vi "oa_Draw Grids and Plot for SCL Plot.vi"(5 "shaft center line settings":T3={"cartesian grid cosmetics"={"line color"=39168, "text color"=65280, "tick length(3)"=3, "crossing axes"=FALSE, "visible grid?"=TRUE}, "XY plot cosmetics"={"plot color"=16776960, "XY plot type"=enum."connected points", "baseline"=0.0}, "desired font(Application)"=enum."Application Font", "[user-specified font]"={"Font Name:"="", "Size"=0, "Strikeout?"=FALSE, "Italic?"=FALSE, "Underline?"=FALSE, "Outline?"=FALSE, "Shadow?"=FALSE, "Bold?"=FALSE}} {"XY plot cosmetics"."baseline" format="%0.2f"}, 6 "shaft rotating direction":u16(ring) items=["CCW", "CW"], 7 "picture \ndimensions (w,h)":cluster{"width":u32, "height":u32}, 8 "error in (no error)":errorcluster, 9 "scale":T1, 10 "DC Gap":cluster{"X":dbl[], "Y":dbl[]}[](array[cluster]) {"Y" format="%.2f"; "X" format="%.2f"}, 11 "picture":picture) -> (0 "error out":errorcluster, 1 "y scale factors":cluster{"a":dbl, "b":dbl, "log?":bool} {"b" format="%0.2f"; "a" format="%0.2f"}, 2 "x scale factors":cluster{"a":dbl, "b":dbl, "log?":bool} {"b" format="%0.2f"; "a" format="%0.2f"}, 3 "new picture":picture)   [LabVIEW 2017]
uses:
  <vilib>/picture/cartesn2.llb/XY Plot Type.ctl
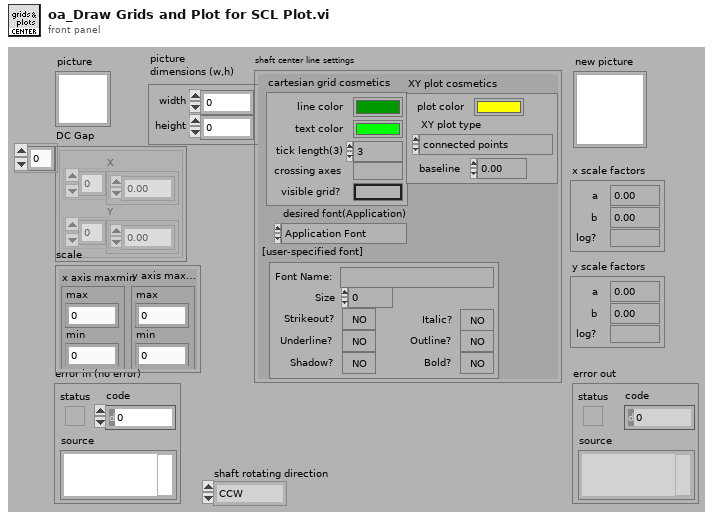
[diagram p1: front panel]
types:
  T1 = cluster{"x axis maxmin":cluster{"max":dbl, "min":dbl}, "y axis maxmin":cluster{"max":dbl, "min":dbl}}
  T2 = typedef "XY Plot Type.ctl" = enum16{"points", "squares", "circles", "connected points", "connected squares", "connected circles", "comb plot", "sized scatter plot", "sized-colored scatter plot", "min-max lines"}
  T3 = cluster{"cartesian grid cosmetics":cluster{"line color":u32, "text color":u32, "tick length(3)":i16, "crossing axes":bool, "visible grid?":bool}, "XY plot cosmetics":cluster{"plot color":u32, "XY plot type":T2, "baseline":dbl}, "desired font(Application)":enum16{"User-specified Font", "Application Font", "System Font", "Dialog Font"}, "[user-specified font]":cluster{"Font Name:":string, "Size":i16, "Strikeout?":bool, "Italic?":bool, "Underline?":bool, "Outline?":bool, "Shadow?":bool, "Bold?":bool}}
  T4 = cluster{"x minimum":dbl, "x maximum":dbl, "x log?":bool, "x precision":u8, "x format":enum8{"Decimal", "Scientific", "Engineering", "Binary", "Octal", "Hex"}, "y minimum":dbl, "y maximum":dbl, "y log?":bool, "y precision":u8, "y format":enum8{"Decimal", "Scientific", "Engineering", "Binary", "Octal", "Hex"}}
  T5 = enum8{"Decimal", "Scientific", "Engineering", "Binary", "Octal", "Hex"}
  T6 = cluster{"line color":u32, "text color":u32, "tick length(3)":i16, "crossing axes":bool, "visible grid?":bool}
  T7 = cluster{"plot color":u32, "XY plot type":T2, "baseline":dbl}
  T8 = enum16{"User-specified Font", "Application Font", "System Font", "Dialog Font"}
  T9 = cluster{"Font Name:":string, "Size":i16, "Strikeout?":bool, "Italic?":bool, "Underline?":bool, "Outline?":bool, "Shadow?":bool, "Bold?":bool}
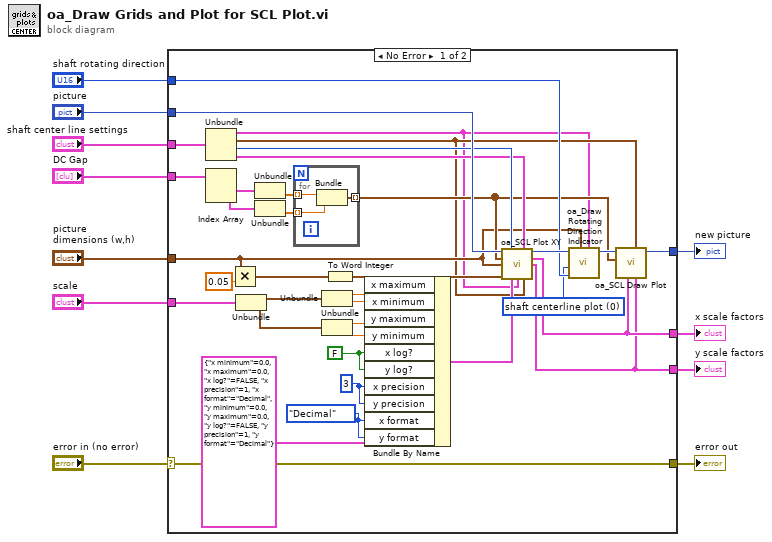
[diagram p0: block diagram]
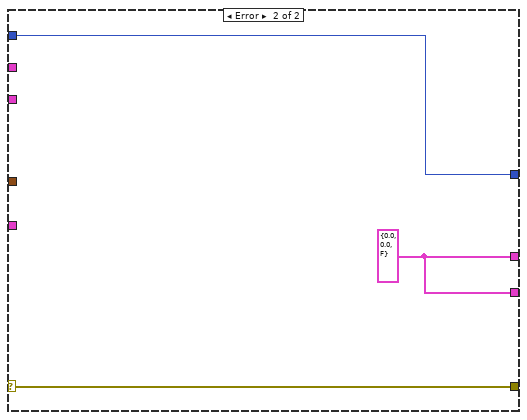
[diagram p2: hidden frame]
diagram:
  n1 = case shown="No Error" "error in (no error)" {
    selector: "error in (no error)" -> [w45 w53]
    tunnel: [w45 w53] -> w10
    tunnel: "picture" -> [w47 w52]
    tunnel: "shaft center line settings" -> [w46 _]
    tunnel: "picture \ndimensions (w,h)" -> [w17 _]
    tunnel: [w19 w52] -> w6
    tunnel: "DC Gap" -> [w44 _]
    tunnel: "scale" -> [w36 _]
    tunnel: "shaft rotating direction" -> [w21 _]
    tunnel: [w15 w51] -> w2
    tunnel: [w14 w51] -> w1
    frame No Error {
      w27 = T5."Decimal" ("x format")
      w28 = u8 3 ("x precision")
      w12 = u16 0 items=["shaft centerline plot", "polar plot"] ("plot type")
      w29 = FALSE ("x log?")
      n2 = Unbundle(w46) -> ("cartesian grid cosmetics"=w13:T6, "XY plot cosmetics"=w16:T7, "desired font(Application)"=w39:T8, "[user-specified font]"=w38:T9)
      n3 = Index Array(array=w44) -> (element #1=w43:cluster{"X":dbl[], "Y":dbl[]}, element #2=w42:cluster{"X":dbl[], "Y":dbl[]})  [unwired: 2 in]
      n4 = Multiply(x=w17, y=0.05) -> (x*y=w24:cluster{"width":dbl, "height":dbl})
      n5 = Unbundle(w36) -> ("x axis maxmin"=w35:cluster{"max":dbl, "min":dbl}, "y axis maxmin"=w33:cluster{"max":dbl, "min":dbl})
      n6 = Unbundle(w43) -> ("Y"=w41:dbl[])  [unwired: 1 out]
      n7 = Unbundle(w42) -> ("Y"=w40:dbl[])  [unwired: 1 out]
      n8 = for {
        tunnel: w41 -> [w50] mode=indexing
        tunnel: w40 -> [w49] mode=indexing
        tunnel: [w48] -> w18 mode=indexing
        n9 = Bundle(w50, w49) -> (w48:cluster{dbl, dbl})  [unwired: 1 in]
      }
      n10 = Unbundle(w35) -> ("max"=w34:dbl, "min"=w32:dbl)
      n11 = Unbundle(w33) -> ("max"=w31:dbl, "min"=w30:dbl)
      n12 = To Word Integer(number=w24) -> (16bit integer=w23:cluster{"width":i16, "height":i16})
      n13 = Bundle By Name(cluster=T4 {"x minimum"=0.0, "x maximum"=0.0, "x log?"=FALSE, "x precision"=1, "x format"=enum."Decimal", "y minimum"=0.0, "y maximum"=0.0, "y log?"=FALSE, "y precision"=1, "y format"=enum."Decimal"} ("cartesian axis attributes"), "x maximum"=w34, "x minimum"=w32, "y maximum"=w31, "y minimum"=w30, "x log?"=w29, "y log?"=w29, "x precision"=w28, "y precision"=w28, "x format"=w27, "y format"=w27) -> (w26:T4)
      n14 = call <vilib>:"oa_SCL Plot XY.vi"("picture"=w47, "desired font(Application)"=w39, "[user-specified font]"=w38, "data"=w18, "dimensions (w,h)"=w17, "top left point(0, 0)"=w23, "cartesian axis attributes"=w26, "cartesian grid cosmetics"=w13, "XY plot cosmetics"=w16) -> ("new picture"=w22:picture, "x scale factors"=w15:cluster{"a":dbl, "b":dbl, "log?":bool}, "y scale factors"=w14:cluster{"a":dbl, "b":dbl, "log?":bool})  [unwired: 4 in]
      n15 = call <vilib>:"oa_Draw Rotating Direction Indicator.vi"("cartesian grid cosmetics"=w13, "picture \ndimensions (w,h)"=w17, "shaft rotating direction"=w21, "plot type"=w12, "picture"=w22) -> ("new picture"=w20:picture)  [unwired: 6 in]
      n16 = call <vilib>:"oa_SCL Draw Plot.vi"("y scale factors"=w14, "XY plot cosmetics"=w16, "x scale factors"=w15, "data"=w18, "picture"=w20) -> ("new picture"=w19:picture)  [unwired: 6 in]
    }
    frame Error {
      w51 = cluster{"a":dbl, "b":dbl, "log?":bool} {"a"=0.0, "b"=0.0, "log?"=FALSE} ("x scale factors")
    }
  }
  "error out" <- w10
  "new picture" <- w6
  "x scale factors" <- w2
  "y scale factors" <- w1
